vi "Pcre2SubstringByNumber8.vi"(8 "error in":errorcluster, 10 "Number":i32, 11 "pMatchData":u64 format="%.0x") -> (0 "error out":errorcluster, 2 "Substring":string, 3 "pMatchData":u64 format="%.0x")   [LabVIEW 2021, in "libpcre2-8.lvlib"]
uses:
  libpcre2-8.lvlib
  Pcre2ErrorNull.vi
  Pcre2FnkCallError.vi
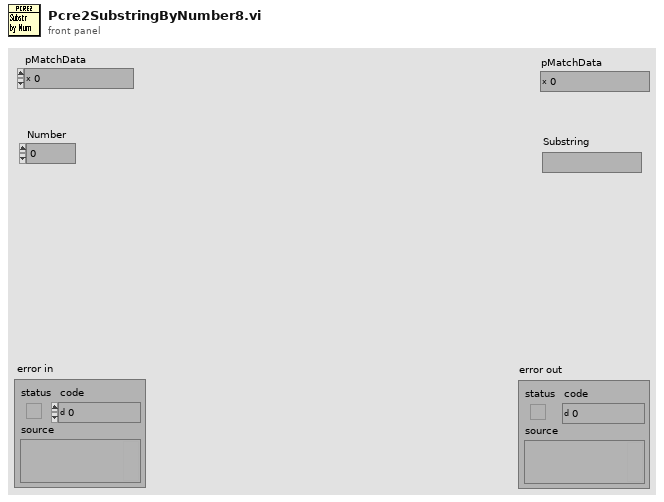
[diagram p1: front panel]
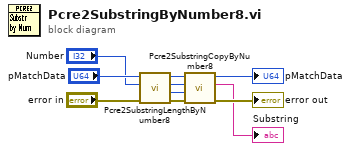
[diagram p0: block diagram]
diagram:
  n1 = call "Pcre2SubstringLengthByNumber8.vi"("error in"="error in", "Number"="Number", "pMatchData"="pMatchData") -> ("error out"=w5:errorcluster, "Length"=w6:u64, "Number"=w7:i32, "pMatchData"=w8:u64)  [unwired: 5 in]
  n2 = call "Pcre2SubstringCopyByNumber8.vi"("error in"=w5, "Length"=w6, "Number"=w7, "pMatchData"=w8) -> ("error out"=→"error out":errorcluster, "Substring"=→"Substring":string, "pMatchData"=→"pMatchData":u64)  [unwired: 5 in]
